vi "config_thcd401.vi"(10 "port":u16=101, 11 "address":string="192.168.24.186") -> (0 "error out":errorcluster)   [LabVIEW 2019]
panel:
  out "status_init":bool
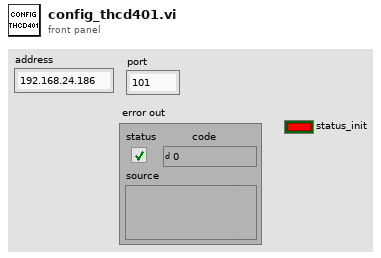
[diagram p1: front panel]
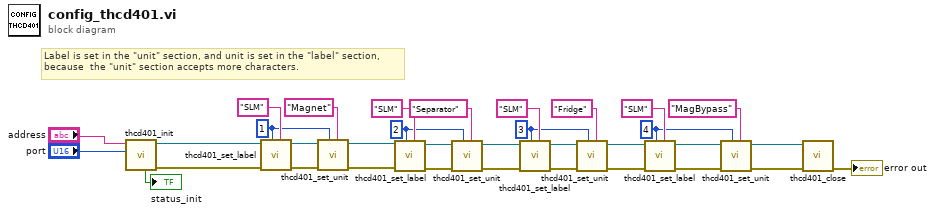
[diagram p0: block diagram]
diagram:
  w10 = u8 4 ("channel")
  w15 = u8 3 ("channel")
  w20 = u8 2 ("channel")
  w25 = u8 1 ("channel")
  # "Label is set in the \"unit\" section, and unit is set in the \"label\" section,\nbecause  the \"unit\" section accepts more characters."
  n1 = call "thcd401_init.vi"("port"="port", "address"="address") -> ("error out"=w29:errorcluster, "conn_id"=w31:refnum<k5>, "status"=→"status_init":bool)  [unwired: 7 in]
  n2 = call "thcd401_set_label.vi"("label"="SLM", "channel"=w25, "error in"=w29, "conn_id_in"=w31) -> ("error out"=w26:errorcluster, "conn_id_out"=w27:refnum<k5>)  [unwired: 5 in, 1 out]
  n3 = call "thcd401_set_unit.vi"("unit"="Magnet", "channel"=w25, "error in"=w26, "conn_id_in"=w27) -> ("error out"=w7:errorcluster, "conn_id_out"=w8:refnum<k5>)  [unwired: 5 in, 1 out]
  n4 = call "thcd401_set_label.vi"("label"="SLM", "channel"=w20, "error in"=w7, "conn_id_in"=w8) -> ("error out"=w21:errorcluster, "conn_id_out"=w22:refnum<k5>)  [unwired: 5 in, 1 out]
  n5 = call "thcd401_set_unit.vi"("unit"="Separator", "channel"=w20, "error in"=w21, "conn_id_in"=w22) -> ("error out"=w6:errorcluster, "conn_id_out"=w5:refnum<k5>)  [unwired: 5 in, 1 out]
  n6 = call "thcd401_set_label.vi"("label"="SLM", "channel"=w15, "error in"=w6, "conn_id_in"=w5) -> ("error out"=w16:errorcluster, "conn_id_out"=w17:refnum<k5>)  [unwired: 5 in, 1 out]
  n7 = call "thcd401_set_unit.vi"("unit"="Fridge", "channel"=w15, "error in"=w16, "conn_id_in"=w17) -> ("error out"=w3:errorcluster, "conn_id_out"=w4:refnum<k5>)  [unwired: 5 in, 1 out]
  n8 = call "thcd401_set_label.vi"("label"="SLM", "channel"=w10, "error in"=w3, "conn_id_in"=w4) -> ("error out"=w11:errorcluster, "conn_id_out"=w12:refnum<k5>)  [unwired: 5 in, 1 out]
  n9 = call "thcd401_set_unit.vi"("unit"="MagBypass", "channel"=w10, "error in"=w11, "conn_id_in"=w12) -> ("error out"=w1:errorcluster, "conn_id_out"=w2:refnum<k5>)  [unwired: 5 in, 1 out]
  n10 = call "thcd401_close.vi"("error in"=w1, "conn_id"=w2) -> ("error out"=→"error out":errorcluster)  [unwired: 8 in, 1 out]
